vi "Meandr_FPGA.vi"() -> ()   [LabVIEW 2018]
uses:
  <vilib>/userdefined/High Color/nirio_resource_hc.ctl
  <vilib>/FPGAPlugInAG/PXI-7951R/niLvFpga_Open_PXI-7951R.vi
  <vilib>/FPGAPlugInAG/PXI-7951R/niLvFpga_Reset_PXI-7951R.vi
  <vilib>/FPGAPlugInAG/PXI-7951R/niLvFpga_Run_PXI-7951R.vi
  <vilib>/Utility/error.llb/Error Cluster From Error Code.vi
  <vilib>/rvi/errors/niLvFpgaAdjustHostInterfaceError.vi
  <vilib>/FPGAPlugInAG/PXI-7951R/niLvFpga_Close_PXI-7951R.vi
  <vilib>/rvi/interface/nirviOpenFPGA/nirviOpenFPGA.xnode
  FPGA Bitfiles/StudyFPGAtarget_FPGATarget_Miganie_-7uDoRG8yQg.lvbitx
  <vilib>/rvi/interface/nirviMethod/nirviMethod.xnode
  <vilib>/rvi/interface/nirviReadWriteControl/nirviReadWriteControl.xnode
  <vilib>/rvi/interface/nirviCloseFPGA/nirviCloseFPGA.xnode
  NiFpgaLv.dll
panel:
  in  "Output enabled CH0 3":bool
  in  "Output enabled CH0 2":bool
  in  "Output enabled CH0":bool
  out "U CH0.2, В":dbl=-0.0007980724207969535
  out "U CH0.1, В":dbl=0.0005291359057392869
  out "U CH0.0, В":dbl=0.00019408818597683764
  out "error out (4110)":errorcluster
  out "I CH0.2, A":dbl=-3.736887207591525e-07
  out "I CH0.1, A":dbl=1.3536171067546387e-06
  out "I CH0.0, A":dbl=0.0001493149910500613
  in  "Скважность":dbl=2.0
  out "Real time without, нс":i16=100
  out "Real time, нс":i16=100
  in  "Active bits":i16=253 format="%b"
  in  "Voltage level CH1":dbl=3.0
  in  "Остановка target":bool
  in  "Время импульса, нс":i16=100
  in  "Current limit CH1":dbl=0.7 format="%#_13g"
  in  "Current limit CH2":dbl=0.1 format="%#_13g"
  in  "Stop Power":bool
  in  "Voltage level CH0":dbl=1.0 format="%#_13g"
  in  "Voltage level CH2":dbl=-1.0 format="%#_13g"
  in  "Current limit CH0":dbl=0.1 format="%#_13g"
  in  "Power Resource":refnum<k15>="PXI1Slot3"
  out "error out (FPGA)":errorcluster
  in  "resource name":T1="PXI1Slot2" caption="RIO Device"
  # "Ток"
  # "Напряжение"
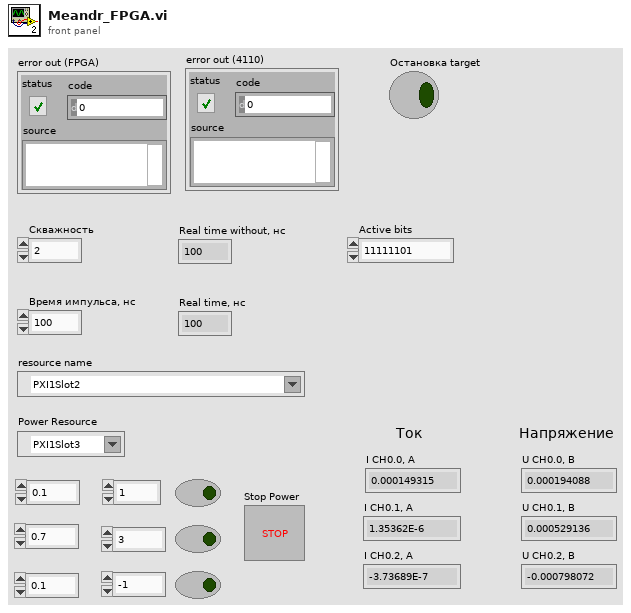
[diagram p1: front panel]
types:
  T1 = typedef "nirio_resource_hc.ctl" = tag
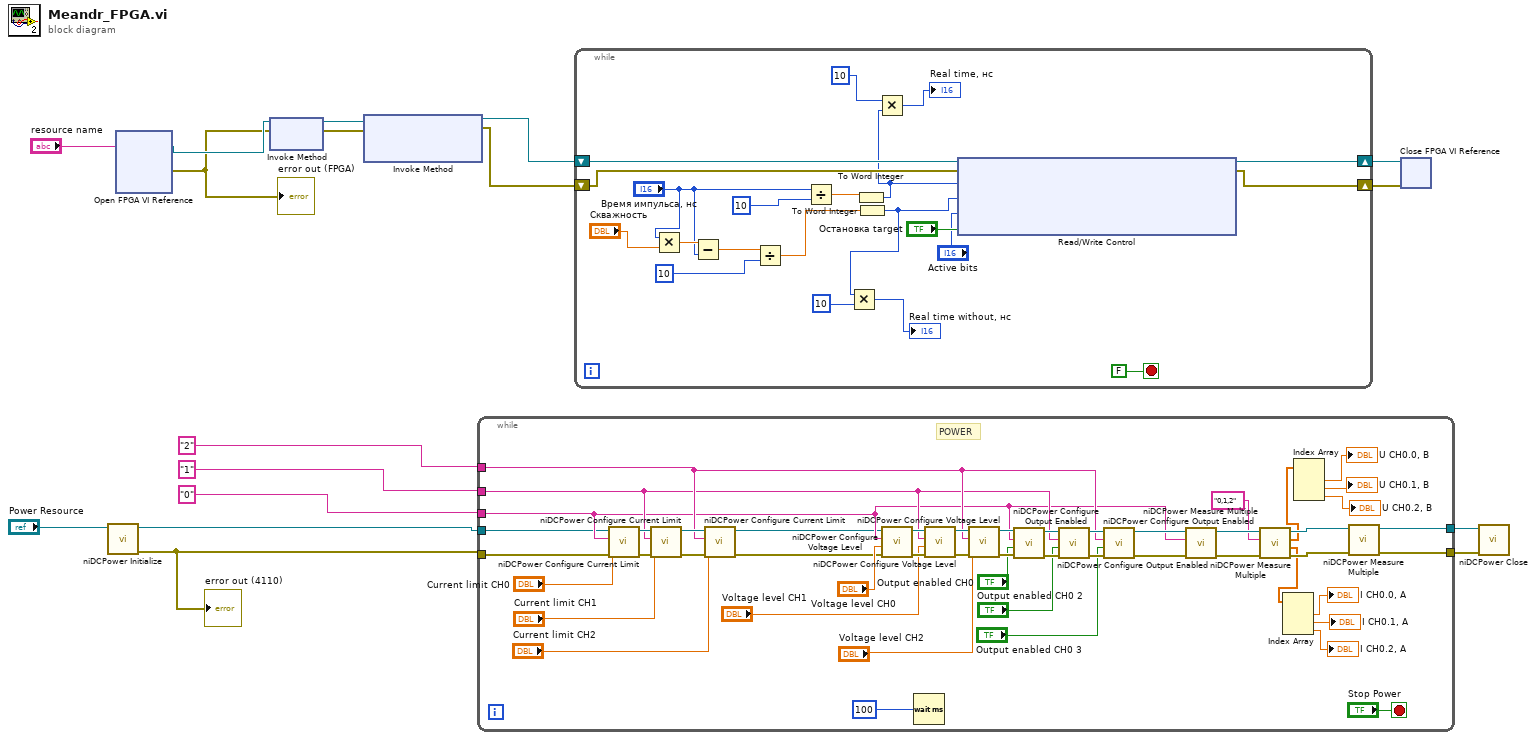
[diagram p0: block diagram]
diagram:
  n1 = call <instrlib>:"niDCPower Initialize.vi"("resource name"="Power Resource") -> ("error out"=w1:errorcluster, "instrument handle out"=w2:refnum<k15>)  [unwired: 3 in, 6 out]
  "error out (4110)" <- w1
  n2 = xnode "Open FPGA VI Reference"("resource name"="resource name") -> ("FPGA VI Reference Out"=w16:refnum<k20>, "error out"=w15:errorcluster)  [unwired: 1 in]
  "error out (FPGA)" <- w15
  n3 = xnode "Invoke Method"("FPGA VI Reference In"=w16, "error in"=w15) -> ("FPGA VI Reference Out"=w12:refnum<k20>, "error out"=w11:errorcluster)
  n4 = xnode ("Invoke Method")("FPGA VI Reference In"=w12, "error in"=w11) -> ("FPGA VI Reference Out"=w3:refnum<k20>, "error out"=w4:errorcluster)  [unwired: 1 in]
  n5 = while {
    tunnel: "0" ("Channel name") -> [w28]
    tunnel: [w46] -> w9
    tunnel: [w49] -> w8
    tunnel: "1" -> [w30]
    tunnel: "2" -> [w31]
    tunnel: w1 -> [w29]
    tunnel: w2 -> [w27]
    stop <- "Stop Power" stop-if-true
    # "POWER"
    n6 = call <instrlib>:"niDCPower Configure Current Limit.vi"("error in (no error)"=w29, "current limit"="Current limit CH0", "channel name"=w28, "instrument handle"=w27) -> ("error out"=w35:errorcluster, "instrument handle out"=w33:refnum<k15>)  [unwired: 6 in]
    n7 = call <instrlib>:"niDCPower Configure Current Limit.vi"("error in (no error)"=w35, "current limit"="Current limit CH1", "channel name"=w30, "instrument handle"=w33) -> ("error out"=w36:errorcluster, "instrument handle out"=w34:refnum<k15>)  [unwired: 6 in]
    n8 = call <instrlib>:"niDCPower Configure Current Limit.vi"("error in (no error)"=w36, "current limit"="Current limit CH2", "channel name"=w31, "instrument handle"=w34) -> ("error out"=w26:errorcluster, "instrument handle out"=w25:refnum<k15>)  [unwired: 6 in]
    n9 = call <instrlib>:"niDCPower Configure Voltage Level.vi"("error in (no error)"=w26, "voltage level"="Voltage level CH0", "channel name"=w28, "instrument handle"=w25) -> ("error out"=w63:errorcluster, "instrument handle out"=w59:refnum<k15>)  [unwired: 6 in]
    n10 = Wait (ms)(milliseconds to wait=u32 100) -> ()  [unwired: 1 out]
    n11 = call <instrlib>:"niDCPower Configure Voltage Level.vi"("error in (no error)"=w63, "voltage level"="Voltage level CH1", "channel name"=w30, "instrument handle"=w59) -> ("error out"=w62:errorcluster, "instrument handle out"=w58:refnum<k15>)  [unwired: 6 in]
    n12 = call <instrlib>:"niDCPower Configure Voltage Level.vi"("error in (no error)"=w62, "voltage level"="Voltage level CH2", "channel name"=w31, "instrument handle"=w58) -> ("error out"=w61:errorcluster, "instrument handle out"=w60:refnum<k15>)  [unwired: 6 in]
    n13 = call <instrlib>:"niDCPower Configure Output Enabled.vi"("error in (no error)"=w61, "output enabled"="Output enabled CH0", "channel name"=w28, "instrument handle"=w60) -> ("error out"=w56:errorcluster, "instrument handle out"=w57:refnum<k15>)  [unwired: 6 in]
    n14 = call <instrlib>:"niDCPower Configure Output Enabled.vi"("error in (no error)"=w56, "output enabled"="Output enabled CH0 2", "channel name"=w30, "instrument handle"=w57) -> ("error out"=w55:errorcluster, "instrument handle out"=w54:refnum<k15>)  [unwired: 6 in]
    n15 = call <instrlib>:"niDCPower Configure Output Enabled.vi"("error in (no error)"=w55, "output enabled"="Output enabled CH0 3", "channel name"=w31, "instrument handle"=w54) -> ("error out"=w52:errorcluster, "instrument handle out"=w53:refnum<k15>)  [unwired: 6 in]
    n16 = call <instrlib>:"niDCPower Measure Multiple.vi"("error in (no error)"=w52, "channel name"=w28, "instrument handle"=w53) -> ("error out"=w48:errorcluster, "instrument handle out"=w51:refnum<k15>)  [unwired: 5 in, 2 out]
    n17 = call <instrlib>:"niDCPower Measure Multiple.vi"("error in (no error)"=w48, "channel name"="0,1,2", "instrument handle"=w51) -> ("error out"=w47:errorcluster, "current measurements"=w42:dbl[], "voltage measurements"=w24:dbl[], "instrument handle out"=w50:refnum<k15>)  [unwired: 5 in]
    n18 = Index Array(array=w42) -> (element #1=→"I CH0.0, A":dbl, element #2=→"I CH0.1, A":dbl, element #3=→"I CH0.2, A":dbl)  [unwired: 3 in]
    n19 = Index Array(array=w24) -> (element #1=→"U CH0.0, В":dbl, element #2=→"U CH0.1, В":dbl, element #3=→"U CH0.2, В":dbl)  [unwired: 3 in]
    n20 = call <instrlib>:"niDCPower Measure Multiple.vi"("error in (no error)"=w47, "instrument handle"=w50) -> ("error out"=w46:errorcluster, "instrument handle out"=w49:refnum<k15>)  [unwired: 6 in, 2 out]
  }
  n21 = while {
    shift-right: [w84] -> w14
    shift-left: w3 -> [w86]
    shift-right: [w83] -> w13
    shift-left: w4 -> [w85]
    stop <- FALSE stop-if-true
    n22 = Multiply(x="Время импульса, нс", y="Скважность") -> (x*y=w75:dbl)
    n23 = Subtract(x=w75, y="Время импульса, нс") -> (x-y=w76:dbl)
    n24 = Divide(x=w76, y=i16 10) -> (x/y=w77:dbl)
    n25 = Divide(x="Время импульса, нс", y=i16 10) -> (x/y=w78:dbl)
    n26 = To Word Integer(number=w78) -> (16bit integer=w71:i16)
    n27 = To Word Integer(number=w77) -> (16bit integer=w69:i16)
    n28 = Multiply(x=w69, y=i16 10) -> (x*y=→"Real time without, нс":i16)
    n29 = Multiply(x=i16 10, y=w71) -> (x*y=→"Real time, нс":i16)
    n30 = xnode "Read/Write Control"("FPGA VI Reference In"=w86, "error in"=w85, "Время импульса, нс"=w71, "Время без импульса"=w69, "Active bits"="Active bits", "stop"="Остановка target") -> ("FPGA VI Reference Out"=w84:refnum<k20>, "error out"=w83:errorcluster)
  }
  n31 = xnode "Close FPGA VI Reference"("FPGA VI Reference In"=w14, "error in"=w13) -> ()  [unwired: 1 out]
  n32 = call <instrlib>:"niDCPower Close.vi"("error in (no error)"=w9, "instrument handle"=w8) -> ()  [unwired: 9 in, 1 out]
